vi "frw_array2csv.vi"(8 "error in":errorcluster, 10 "2Darray":dbl[][](array[numeric]), 11 "file path in":path) -> (0 "error out":errorcluster, 3 "path out":path)   [LabVIEW 2013]
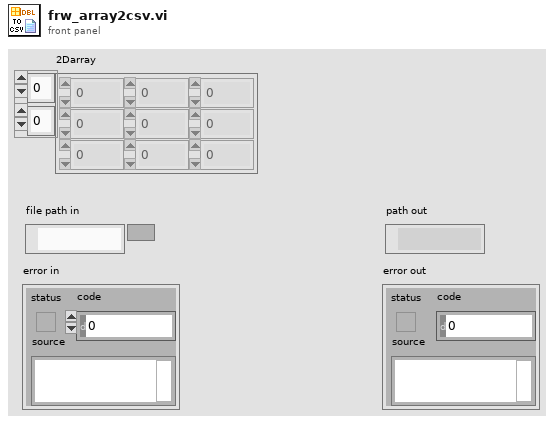
[diagram p1: front panel]
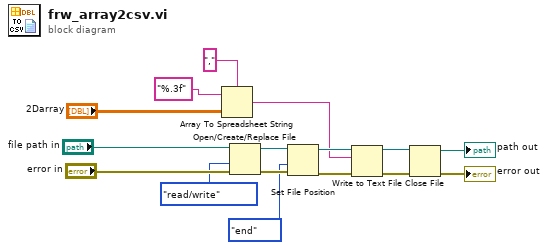
[diagram p0: block diagram]
diagram:
  n1 = Array To Spreadsheet String(delimiter (Tab)=",", array="2Darray", 3:"%.3f" ("format string")) -> (spreadsheet string=w1:string)
  n2 = Open/Create/Replace File(file path (use dialog)="file path in", error in="error in", access (0:read/write)=enum16{"read/write", "read-only", "write-only"}."read/write") -> (refnum out=w9:refnum<file>, error out=w11:errorcluster)  [unwired: 1 in, 3 out]
  n3 = Set File Position(refnum=w9, from (0:start)=enum16{"start", "end", "current"}."end", error in=w11) -> (refnum out=w8:refnum<file>, error out=w7:errorcluster)  [unwired: 1 in]
  n4 = Write to Text File(file (use dialog)=w8, text=w1, error in=w7) -> (refnum out=w5:refnum<file>, error out=w6:errorcluster)  [unwired: 2 out]
  n5 = Close File(refnum=w5, error in=w6) -> (path=→"path out":path, error out=→"error out":errorcluster)
